vi "灰度曲线.vi"() -> ()   [LabVIEW 2018]
uses:
  <vilib>/vision/NI_Vision_Development_Module.lvlib
panel:
  out "error out":errorcluster
  out "波形图":cluster{"x0":sgl, "dx":sgl, "Pixels Line":sgl[]}(graph)
  out "Image":T1(plugin-control)
  in  "路径":path
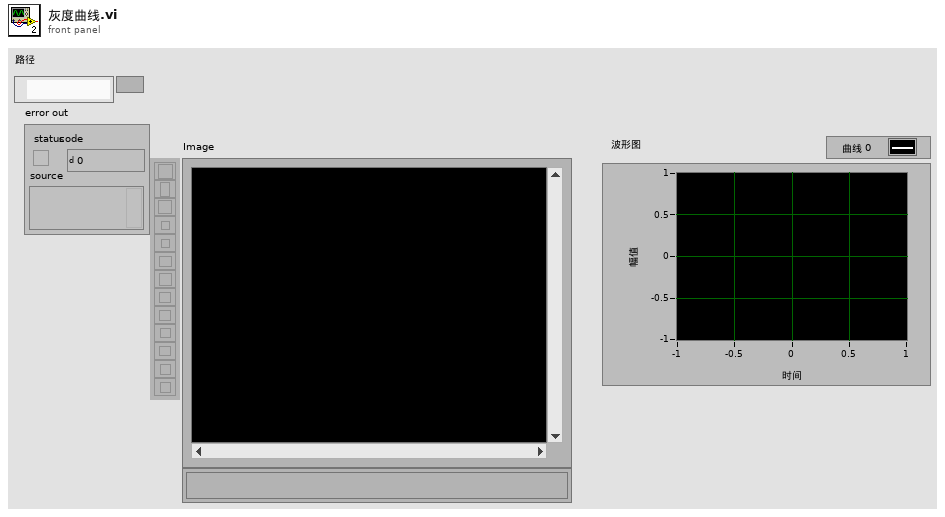
[diagram p1: front panel]
types:
  T1 = typedef "IMAQ Image.ctl" = refnum<image>
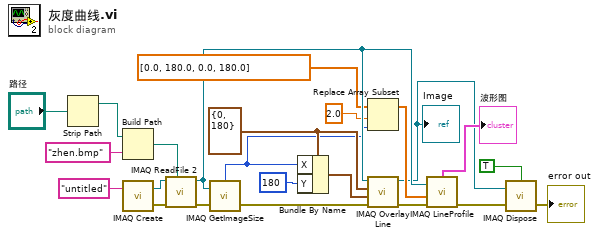
[diagram p0: block diagram]
diagram:
  w14 = cluster{"X":i32, "Y":i32} {"X"=0, "Y"=180} ("Start Point")
  n1 = Strip Path(path="路径") -> (stripped path=w22:path)  [unwired: 1 out]
  n2 = Build Path(base path=w22, name or relative path="zhen.bmp" ("名称或相对路径")) -> (appended path=w17:path)
  n3 = call "IMAQ Create"("Image Name"="untitled") -> ("New Image"=w19:T1, "error out"=w18:errorcluster)  [unwired: 4 in]
  n4 = call "IMAQ ReadFile 2"("File Path"=w17, "error in (no error)"=w18, "Image"=w19) -> ("error out"=w16:errorcluster, "Image Out"=w11:T1)  [unwired: 4 in, 3 out]
  n5 = call "IMAQ GetImageSize"("Image"=w11, "error in (no error)"=w16) -> ("X Resolution"=w7:i32, "error out"=w15:errorcluster)  [unwired: 2 in, 1 out]
  n6 = Bundle By Name(cluster=w14, "X"=w7, "Y"=180) -> (w12:cluster{"X":i32, "Y":i32})
  n7 = Replace Array Subset(array=dbl[] [0.0, 180.0, 0.0, 180.0] ("数组"), new element=w7, index=2.0 ("新元素/子数组")) -> (w6:dbl[])
  n8 = call "IMAQ Overlay Line"("error in (no error)"=w15, "End Point"=w12, "Start Point"=w14, "Image"=w11) -> ("error out"=w10:errorcluster, "Image Out"=w4:T1)  [unwired: 6 in]
  "Image" <- w4
  n9 = call "IMAQ LineProfile"("error in (no error)"=w10, "Line Coordinates"=w6, "Image"=w11) -> ("error out"=w3:errorcluster, "Line Graph"=→"波形图":cluster{"x0":sgl, "dx":sgl, "Pixels Line":sgl[]})  [unwired: 2 in, 2 out]
  n10 = call "IMAQ Dispose"("All Images? (No)"=TRUE, "Image"=w4, "error in (no error)"=w3) -> ("error out"=→"error out":errorcluster)  [unwired: 3 in]
